vi "CreateScanPattern.vi"(3 "Point Spacing":dbl, 4 "Number of Points":u8, 5 "Pattern":T1(ring)) -> (0 "Radius":dbl, 1 "Y coordinates":dbl[](array[numeric]), 2 "X coordinates":dbl[](array[numeric]))   [LabVIEW 2011]
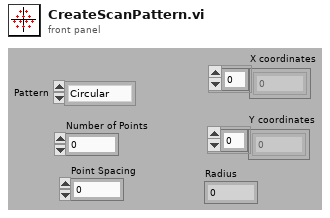
[diagram p1: front panel]
types:
  T1 = enum8{"Circular", "Square", "Hexagonal", "FilledSquare"}
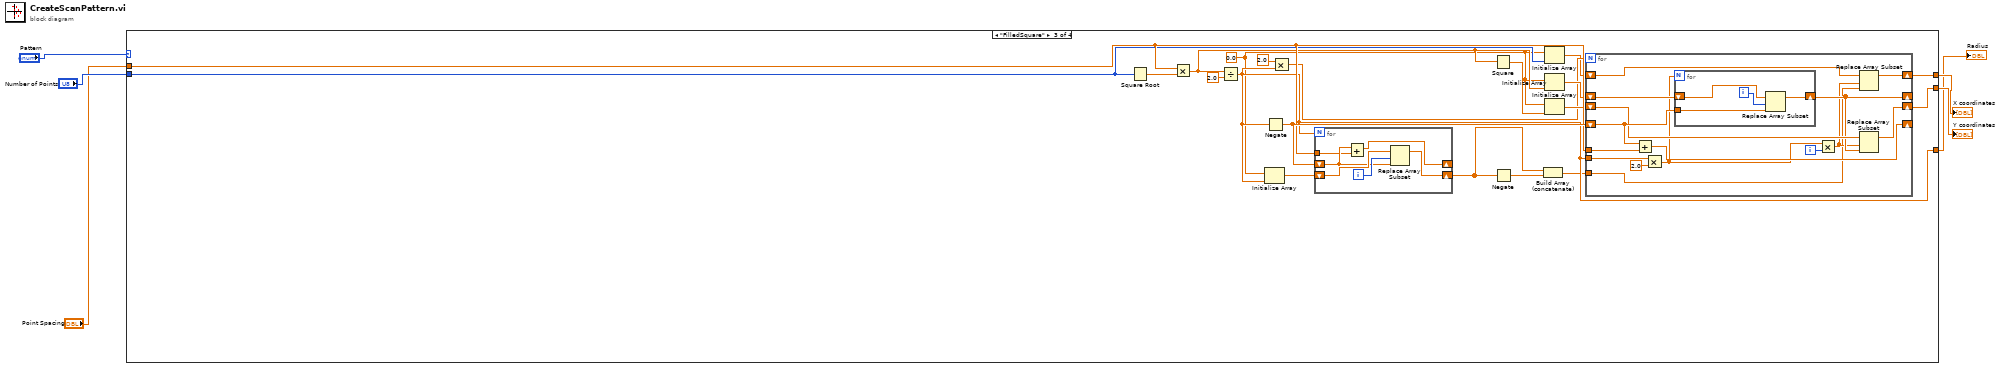
[diagram p0: block diagram]
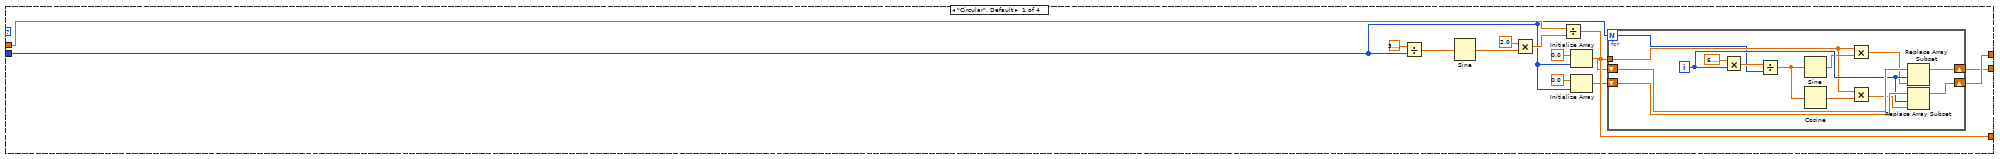
[diagram p2: hidden frame]
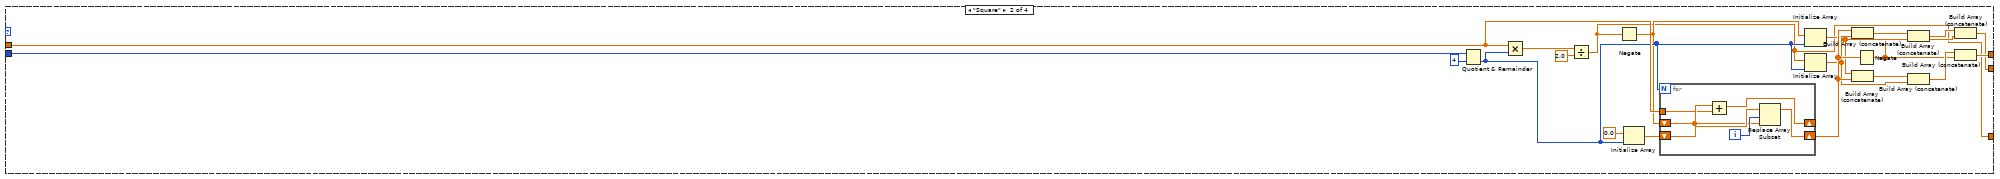
[diagram p3: hidden frame]
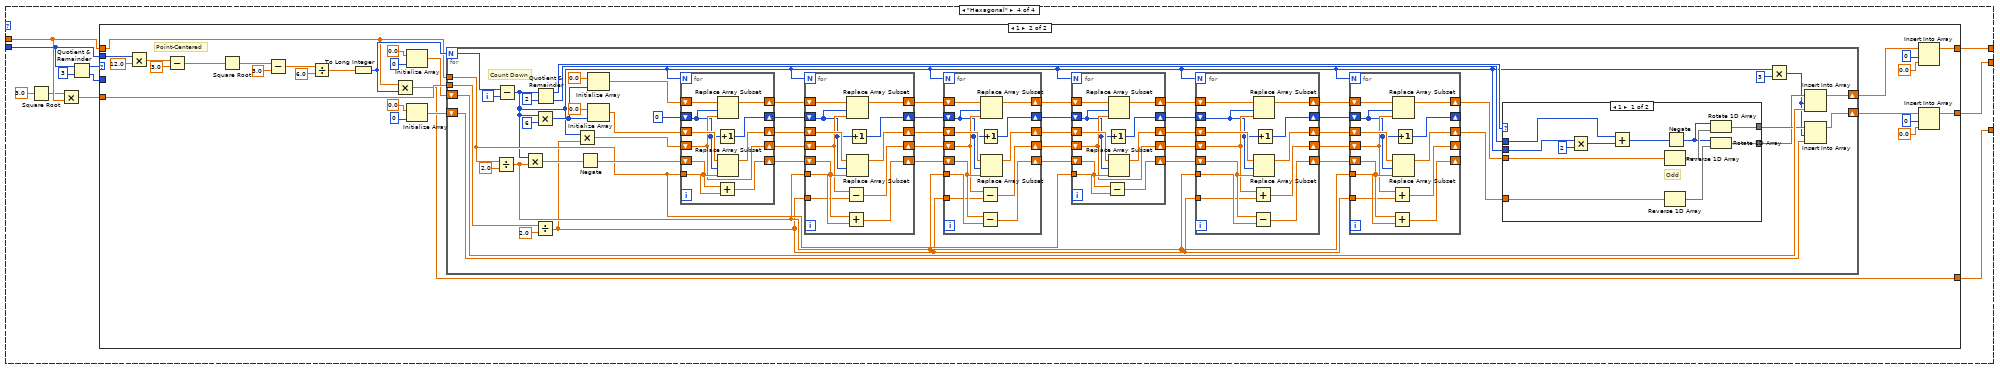
[diagram p4: hidden frame]
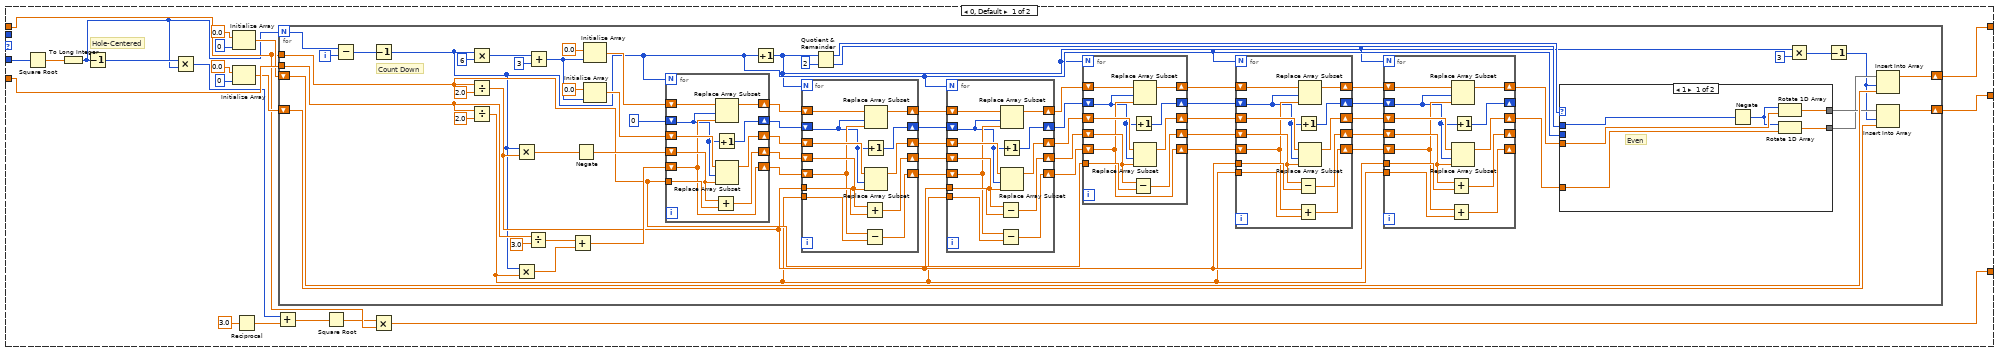
[diagram p5: hidden frame]
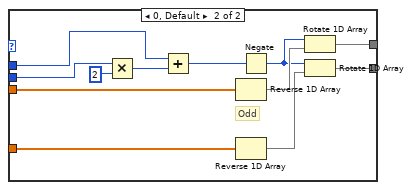
[diagram p6: hidden frame]
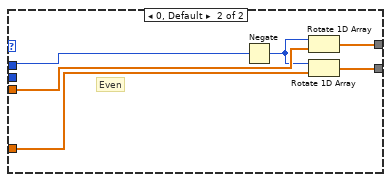
[diagram p7: hidden frame]
diagram:
  n1 = case shown="\"FilledSquare\"" "Pattern" {
    tunnel: "Point Spacing" -> [w15 w48 w75 w112]
    tunnel: "Number of Points" -> [w7 w54 w66 w107]
    tunnel: [w14 w43 w61 w109] -> w4
    tunnel: [w13 w40 w64 w108] -> w3
    tunnel: [w12 w35 w68 w106] -> w2
    frame "Circular", Default {
      n2 = Divide(x=3.141592653589793, y=w7) -> (x/y=w19:dbl)
      n3 = Sine(x=w19) -> (sin(x)=w18:dbl)
      n4 = Multiply(x=2.0, y=w18) -> (x*y=w16:dbl)
      n5 = Divide(x=w15, y=w16) -> (x/y=w12:dbl)
      n6 = Initialize Array(0.0 ("element"), w7) -> (w9:dbl[])
      n7 = Initialize Array(0.0 ("element"), w7) -> (w8:dbl[])
      n8 = for {
        N: w7 -> [w21]
        shift-right: [w28] -> w13
        shift-left: w9 -> [w33]
        shift-right: [w27] -> w14
        shift-left: w8 -> [w34]
        tunnel: w12 -> [w24]
        i -> [w32]
        n9 = Multiply(x=6.283185307179586, y=w32) -> (x*y=w30:dbl)
        n10 = Divide(x=w30, y=w21) -> (x/y=w29:dbl)
        n11 = Sine(x=w29) -> (sin(x)=w25:dbl)
        n12 = Cosine(x=w29) -> (cos(x)=w26:dbl)
        n13 = Multiply(x=w24, y=w25) -> (x*y=w23:dbl)
        n14 = Multiply(x=w24, y=w26) -> (x*y=w22:dbl)
        n15 = Replace Array Subset(array=w33, new element=w23, index=w32) -> (w28:dbl[])
        n16 = Replace Array Subset(array=w34, new element=w22, index=w32) -> (w27:dbl[])
      }
    }
    frame "Square" {
      n17 = Quotient & Remainder(x=w54, y=u8 4) -> (floor(x/y)=w47:u8)  [unwired: 1 out]
      n18 = Multiply(x=w48, y=w47) -> (x*y=w52:dbl)
      n19 = Divide(x=w52, y=2.0) -> (x/y=w35:dbl)
      n20 = Negate(x=w35) -> (-x=w46:dbl)
      n21 = Initialize Array(0.0 ("element"), w47) -> (w49:dbl[])
      n22 = for {
        N: w47 -> [_]
        shift-right: [w56] -> _
        shift-left: w46 -> [w58]
        shift-right: [w55] -> w39
        shift-left: w49 -> [w60]
        tunnel: w48 -> [w57]
        i -> [w59]
        n23 = Add(x=w58, y=w57) -> (x+y=w56:dbl)
        n24 = Replace Array Subset(array=w60, new element=w58, index=w59) -> (w55:dbl[])
      }
      n25 = Initialize Array(w46, w47) -> (w37:dbl[])
      n26 = Initialize Array(w35, w47) -> (w38:dbl[])
      n27 = Build Array (concatenate)(w39, w38) -> (w42:dbl[])
      n28 = Build Array (concatenate)(w37, w39) -> (w45:dbl[])
      n29 = Negate(x=w39) -> (-x=w36:dbl[])
      n30 = Build Array (concatenate)(w42, w36) -> (w41:dbl[])
      n31 = Build Array (concatenate)(w45, w38) -> (w44:dbl[])
      n32 = Build Array (concatenate)(w41, w37) -> (w40:dbl[])
      n33 = Build Array (concatenate)(w44, w36) -> (w43:dbl[])
    }
    frame "FilledSquare" {
      w65 = 0.0 ("element")
      n34 = Square Root(x=w66) -> (sqrt(x)=w79:dbl)
      n35 = Multiply(x=w75, y=w79) -> (x*y=w70:dbl)
      n36 = Divide(x=w70, y=2.0) -> (x/y=w68:dbl)
      n37 = Initialize Array(w65, w68) -> (w74:dbl[])
      n38 = Negate(x=w68) -> (-x=w76:dbl)
      n39 = Multiply(x=2.0, y=w68) -> (x*y=w67:dbl)
      n40 = for {
        N: w68 -> [_]
        shift-right: [w101] -> _
        shift-left: w76 -> [w103]
        shift-right: [w100] -> w78
        shift-left: w74 -> [w105]
        tunnel: w75 -> [w102]
        i -> [w104]
        n41 = Add(x=w103, y=w102) -> (x+y=w101:dbl)
        n42 = Replace Array Subset(array=w105, new element=w103, index=w104) -> (w100:dbl[])
      }
      n43 = Square(x=w70) -> (x^2=w71:dbl)
      n44 = Negate(x=w78) -> (-x=w77:dbl[])
      n45 = Build Array (concatenate)(w78, w77) -> (w62:dbl[])
      n46 = Initialize Array(w65, w66) -> (w63:dbl[])
      n47 = Initialize Array(w65, w70) -> (w73:dbl[])
      n48 = Initialize Array(w65, w71) -> (w72:dbl[])
      n49 = for {
        N: w67 -> [_]
        tunnel: w68 -> [w91]
        tunnel: w75 -> [w93]
        shift-right: [w94] -> _
        shift-left: w76 -> [w92]
        shift-right: [w87] -> _
        shift-left: w73 -> [w95]
        shift-right: [w88] -> w64
        shift-left: w72 -> [w89]
        shift-right: [w81] -> w61
        shift-left: w63 -> [w84]
        tunnel: w62 -> [w82]
        i -> [w85]
        n50 = Add(x=w92, y=w93) -> (x+y=w94:dbl)
        n51 = Multiply(x=w91, y=2.0) -> (x*y=w86:dbl)
        n52 = for {
          N: w86 -> [_]
          tunnel: w92 -> [w98]
          shift-right: [w96] -> w87
          shift-left: w95 -> [w97]
          i -> [w99]
          n53 = Replace Array Subset(array=w97, new element=w98, index=w99) -> (w96:dbl[])
        }
        n54 = Multiply(x=w86, y=w85) -> (x*y=w83:dbl)
        n55 = Replace Array Subset(array=w84, new element=w82, index=w83) -> (w81:dbl[])
        n56 = Replace Array Subset(array=w89, new element=w87, index=w83) -> (w88:dbl[])
      }
    }
    frame "Hexagonal" {
      n57 = Square Root(x=3.0) -> (sqrt(x)=w111:dbl)
      n58 = Multiply(x=w111, y=w112) -> (x*y=w113:dbl)
      n59 = Quotient & Remainder(x=w107, y=u8 3) -> (x-y*floor(x/y)=w115:u8, floor(x/y)=w110:u8)
      n60 = case shown="1" w115 {
        tunnel: w112 -> [w122 w289]
        tunnel: w113 -> [w130 w311]
        tunnel: w110 -> [w136 _]
        tunnel: [w127 w292] -> w109
        tunnel: [w126 w291] -> w108
        tunnel: w107 -> [_ w308]
        tunnel: [w121 w288] -> w106
        frame 0, Default {
          # "Hole-Centered"
          n61 = Square Root(x=w136) -> (sqrt(x)=w135:dbl)
          n62 = To Long Integer(number=w135) -> (32bit integer=w117:i32)
          n63 = Decrement(x=w117) -> (x-1=w118:i32)
          n64 = Multiply(x=w118, y=w117) -> (x*y=w125:i32)
          n65 = Initialize Array(0.0 ("element"), 0 ("dimension size")) -> (w129:dbl[])
          n66 = Initialize Array(0.0 ("element"), 0 ("dimension size")) -> (w128:dbl[])
          n67 = Reciprocal(x=3.0) -> (1/x=w124:dbl)
          n68 = Add(x=w125, y=w124) -> (x+y=w120:dbl)
          n69 = for {
            N: w117 -> [w155]
            tunnel: w122 -> [w172]
            tunnel: w130 -> [w185]
            shift-right: [w152] -> w127
            shift-left: w129 -> [w153]
            shift-right: [w151] -> w126
            shift-left: w128 -> [w149]
            i -> [w154]
            # "Count Down"
            n70 = Subtract(x=w155, y=w154) -> (x-y=w148:i32)
            n71 = Decrement(x=w148) -> (x-1=w141:i32)
            n72 = Multiply(x=w141, y=6) -> (x*y=w145:i32)
            n73 = Divide(x=w172, y=2.0) -> (x/y=w161:dbl)
            n74 = Divide(x=w185, y=2.0) -> (x/y=w160:dbl)
            n75 = Multiply(x=w141, y=w161) -> (x*y=w183:dbl)
            n76 = Multiply(x=w141, y=w160) -> (x*y=w186:dbl)
            n77 = Divide(x=w185, y=3.0) -> (x/y=w199:dbl)
            n78 = Add(x=w145, y=3) -> (x+y=w144:i32)
            n79 = Add(x=w199, y=w186) -> (x+y=w196:dbl)
            n80 = Negate(x=w183) -> (-x=w197:dbl)
            n81 = Initialize Array(0.0 ("element"), w144) -> (w192:dbl[])
            n82 = Initialize Array(0.0 ("element"), w144) -> (w193:dbl[])
            n83 = for {
              N: w141 -> [_]
              shift-right: [w280] -> w190
              shift-left: w197 -> [w283]
              shift-right: [w281] -> w188
              shift-left: w196 -> [w281]
              shift-right: [w286] -> w191
              shift-left: w193 -> [w287]
              shift-right: [w284] -> w189
              shift-left: w192 -> [w285]
              tunnel: w172 -> [w282]
              shift-right: [w278] -> w187
              shift-left: 0 ("y") -> [w279]
              n84 = Add(x=w283, y=w282) -> (x+y=w280:dbl)
              n85 = Increment(x=w279) -> (x+1=w278:i32)
              n86 = Replace Array Subset(array=w285, new element=w281, index=w279) -> (w284:dbl[])
              n87 = Replace Array Subset(array=w287, new element=w283, index=w279) -> (w286:dbl[])
            }
            n88 = Increment(x=w141) -> (x+1=w140:i32)
            n89 = for {
              N: w140 -> [_]
              shift-right: [w272] -> w180
              shift-left: w190 -> [w273]
              shift-right: [w268] -> w178
              shift-left: w188 -> [w270]
              shift-right: [w276] -> w181
              shift-left: w191 -> [w277]
              shift-right: [w274] -> w179
              shift-left: w189 -> [w275]
              tunnel: w161 -> [w271]
              shift-right: [w266] -> w182
              shift-left: w187 -> [w267]
              tunnel: w160 -> [w269]
              n90 = Add(x=w273, y=w271) -> (x+y=w272:dbl)
              n91 = Subtract(x=w270, y=w269) -> (x-y=w268:dbl)
              n92 = Increment(x=w267) -> (x+1=w266:i32)
              n93 = Replace Array Subset(array=w275, new element=w270, index=w267) -> (w274:dbl[])
              n94 = Replace Array Subset(array=w277, new element=w273, index=w267) -> (w276:dbl[])
            }
            n95 = Quotient & Remainder(x=w140, y=2) -> (x-y*floor(x/y)=w158:i32, floor(x/y)=w150:i32)
            n96 = for {
              N: w141 -> [_]
              shift-right: [w260] -> w175
              shift-left: w180 -> [w261]
              shift-right: [w257] -> w173
              shift-left: w178 -> [w258]
              shift-right: [w264] -> w176
              shift-left: w181 -> [w265]
              shift-right: [w262] -> w174
              shift-left: w179 -> [w263]
              tunnel: w161 -> [w259]
              shift-right: [w254] -> w177
              shift-left: w182 -> [w255]
              tunnel: w160 -> [w256]
              n97 = Subtract(x=w261, y=w259) -> (x-y=w260:dbl)
              n98 = Subtract(x=w258, y=w256) -> (x-y=w257:dbl)
              n99 = Increment(x=w255) -> (x+1=w254:i32)
              n100 = Replace Array Subset(array=w263, new element=w258, index=w255) -> (w262:dbl[])
              n101 = Replace Array Subset(array=w265, new element=w261, index=w255) -> (w264:dbl[])
            }
            n102 = for {
              N: w140 -> [_]
              shift-right: [w248] -> w169
              shift-left: w175 -> [w249]
              shift-right: [w246] -> w167
              shift-left: w173 -> [w246]
              shift-right: [w252] -> w170
              shift-left: w176 -> [w253]
              shift-right: [w250] -> w168
              shift-left: w174 -> [w251]
              tunnel: w172 -> [w247]
              shift-right: [w244] -> w171
              shift-left: w177 -> [w245]
              n103 = Subtract(x=w249, y=w247) -> (x-y=w248:dbl)
              n104 = Increment(x=w245) -> (x+1=w244:i32)
              n105 = Replace Array Subset(array=w251, new element=w246, index=w245) -> (w250:dbl[])
              n106 = Replace Array Subset(array=w253, new element=w249, index=w245) -> (w252:dbl[])
            }
            n107 = for {
              N: w141 -> [_]
              shift-right: [w238] -> w164
              shift-left: w169 -> [w239]
              shift-right: [w234] -> w162
              shift-left: w167 -> [w236]
              shift-right: [w242] -> w165
              shift-left: w170 -> [w243]
              shift-right: [w240] -> w163
              shift-left: w168 -> [w241]
              tunnel: w161 -> [w237]
              shift-right: [w232] -> w166
              shift-left: w171 -> [w233]
              tunnel: w160 -> [w235]
              n108 = Subtract(x=w239, y=w237) -> (x-y=w238:dbl)
              n109 = Add(x=w236, y=w235) -> (x+y=w234:dbl)
              n110 = Increment(x=w233) -> (x+1=w232:i32)
              n111 = Replace Array Subset(array=w241, new element=w236, index=w233) -> (w240:dbl[])
              n112 = Replace Array Subset(array=w243, new element=w239, index=w233) -> (w242:dbl[])
            }
            n113 = for {
              N: w140 -> [_]
              shift-right: [w226] -> _
              shift-left: w164 -> [w227]
              shift-right: [w222] -> _
              shift-left: w162 -> [w224]
              shift-right: [w230] -> w157
              shift-left: w165 -> [w231]
              shift-right: [w228] -> w156
              shift-left: w163 -> [w229]
              tunnel: w161 -> [w225]
              shift-right: [w220] -> _
              shift-left: w166 -> [w221]
              tunnel: w160 -> [w223]
              n114 = Add(x=w227, y=w225) -> (x+y=w226:dbl)
              n115 = Add(x=w224, y=w223) -> (x+y=w222:dbl)
              n116 = Replace Array Subset(array=w229, new element=w224, index=w221) -> (w228:dbl[])
              n117 = Replace Array Subset(array=w231, new element=w227, index=w221) -> (w230:dbl[])
              n118 = Increment(x=w221) -> (x+1=w220:i32)
            }
            n119 = case shown="1" w158 {
              tunnel: w157 -> [w205 w219]
              tunnel: w156 -> [w204 w218]
              tunnel: w141 -> [_ w214]
              tunnel: w150 -> [w203 w213]
              tunnel: [w207 w211] -> w146
              tunnel: [w206 w210] -> w147
              frame 1 {
                # "Even"
                n120 = Negate(x=w203) -> (-x=w202:i32)
                n121 = Rotate 1D Array(1:w204, 2:w202) -> (0:w206:dbl[])
                n122 = Rotate 1D Array(1:w205, 2:w202) -> (0:w207:dbl[])
              }
              frame 0, Default {
                # "Odd"
                n123 = Multiply(x=w214, y=2) -> (x*y=w215:i32)
                n124 = Add(x=w213, y=w215) -> (x+y=w209:i32)
                n125 = Reverse 1D Array(array=w218) -> (reversed array=w212:dbl[])
                n126 = Reverse 1D Array(array=w219) -> (reversed array=w217:dbl[])
                n127 = Negate(x=w209) -> (-x=w208:i32)
                n128 = Rotate 1D Array(1:w212, 2:w208) -> (0:w210:dbl[])
                n129 = Rotate 1D Array(1:w217, 2:w208) -> (0:w211:dbl[])
              }
            }
            n130 = Multiply(x=w140, y=3) -> (x*y=w138:i32)
            n131 = Decrement(x=w138) -> (x-1=w137:i32)
            n132 = Insert Into Array(array=w146, index=w137, new element=w153) -> (w152:dbl[])
            n133 = Insert Into Array(array=w147, index=w137, new element=w149) -> (w151:dbl[])
          }
          n134 = Square Root(x=w120) -> (sqrt(x)=w119:dbl)
          n135 = Multiply(x=w119, y=w122) -> (x*y=w121:dbl)
        }
        frame 1 {
          # "Point-Centered"
          n136 = Multiply(x=w308, y=12.0) -> (x*y=w306:dbl)
          n137 = Subtract(x=w306, y=3.0) -> (x-y=w304:dbl)
          n138 = Square Root(x=w304) -> (sqrt(x)=w303:dbl)
          n139 = Subtract(x=w303, y=3.0) -> (x-y=w301:dbl)
          n140 = Divide(x=w301, y=6.0) -> (x/y=w299:dbl)
          n141 = To Long Integer(number=w299) -> (32bit integer=w290:i32)
          n142 = Multiply(x=w289, y=w290) -> (x*y=w288:dbl)
          n143 = Initialize Array(0.0 ("element"), 0 ("dimension size")) -> (w310:dbl[])
          n144 = Initialize Array(0.0 ("element"), 0 ("dimension size")) -> (w309:dbl[])
          n145 = for {
            N: w290 -> [w330]
            tunnel: w289 -> [w347]
            tunnel: w311 -> [w360]
            shift-right: [w327] -> w294
            shift-left: w310 -> [w328]
            shift-right: [w326] -> w293
            shift-left: w309 -> [w324]
            i -> [w329]
            # "Count Down"
            n146 = Divide(x=w347, y=2.0) -> (x/y=w336:dbl)
            n147 = Subtract(x=w330, y=w329) -> (x-y=w318:i32)
            n148 = Multiply(x=w318, y=w336) -> (x*y=w358:dbl)
            n149 = Multiply(x=w318, y=6) -> (x*y=w320:i32)
            n150 = Divide(x=w360, y=2.0) -> (x/y=w335:dbl)
            n151 = Quotient & Remainder(x=w318, y=2) -> (x-y*floor(x/y)=w333:i32, floor(x/y)=w325:i32)
            n152 = Multiply(x=w318, y=w335) -> (x*y=w316:dbl)
            n153 = Negate(x=w358) -> (-x=w370:dbl)
            n154 = Initialize Array(0.0 ("element"), w320) -> (w366:dbl[])
            n155 = Initialize Array(0.0 ("element"), w320) -> (w367:dbl[])
            n156 = for {
              N: w318 -> [_]
              shift-right: [w451] -> w364
              shift-left: w370 -> [w454]
              shift-right: [w452] -> w362
              shift-left: w316 -> [w452]
              shift-right: [w457] -> w365
              shift-left: w367 -> [w458]
              shift-right: [w455] -> w363
              shift-left: w366 -> [w456]
              tunnel: w347 -> [w453]
              shift-right: [w449] -> w361
              shift-left: 0 ("y") -> [w450]
              n157 = Add(x=w454, y=w453) -> (x+y=w451:dbl)
              n158 = Increment(x=w450) -> (x+1=w449:i32)
              n159 = Replace Array Subset(array=w456, new element=w452, index=w450) -> (w455:dbl[])
              n160 = Replace Array Subset(array=w458, new element=w454, index=w450) -> (w457:dbl[])
            }
            n161 = for {
              N: w318 -> [_]
              shift-right: [w443] -> w355
              shift-left: w364 -> [w444]
              shift-right: [w439] -> w353
              shift-left: w362 -> [w441]
              shift-right: [w447] -> w356
              shift-left: w365 -> [w448]
              shift-right: [w445] -> w354
              shift-left: w363 -> [w446]
              tunnel: w336 -> [w442]
              shift-right: [w437] -> w357
              shift-left: w361 -> [w438]
              tunnel: w335 -> [w440]
              n162 = Subtract(x=w441, y=w440) -> (x-y=w439:dbl)
              n163 = Add(x=w444, y=w442) -> (x+y=w443:dbl)
              n164 = Replace Array Subset(array=w446, new element=w441, index=w438) -> (w445:dbl[])
              n165 = Replace Array Subset(array=w448, new element=w444, index=w438) -> (w447:dbl[])
              n166 = Increment(x=w438) -> (x+1=w437:i32)
            }
            n167 = for {
              N: w318 -> [_]
              shift-right: [w431] -> w350
              shift-left: w355 -> [w432]
              shift-right: [w428] -> w348
              shift-left: w353 -> [w429]
              shift-right: [w435] -> w351
              shift-left: w356 -> [w436]
              shift-right: [w433] -> w349
              shift-left: w354 -> [w434]
              tunnel: w336 -> [w430]
              shift-right: [w425] -> w352
              shift-left: w357 -> [w426]
              tunnel: w335 -> [w427]
              n168 = Subtract(x=w429, y=w427) -> (x-y=w428:dbl)
              n169 = Subtract(x=w432, y=w430) -> (x-y=w431:dbl)
              n170 = Increment(x=w426) -> (x+1=w425:i32)
              n171 = Replace Array Subset(array=w434, new element=w429, index=w426) -> (w433:dbl[])
              n172 = Replace Array Subset(array=w436, new element=w432, index=w426) -> (w435:dbl[])
            }
            n173 = for {
              N: w318 -> [_]
              shift-right: [w419] -> w344
              shift-left: w350 -> [w420]
              shift-right: [w417] -> w342
              shift-left: w348 -> [w417]
              shift-right: [w423] -> w345
              shift-left: w351 -> [w424]
              shift-right: [w421] -> w343
              shift-left: w349 -> [w422]
              tunnel: w347 -> [w418]
              shift-right: [w415] -> w346
              shift-left: w352 -> [w416]
              n174 = Subtract(x=w420, y=w418) -> (x-y=w419:dbl)
              n175 = Increment(x=w416) -> (x+1=w415:i32)
              n176 = Replace Array Subset(array=w422, new element=w417, index=w416) -> (w421:dbl[])
              n177 = Replace Array Subset(array=w424, new element=w420, index=w416) -> (w423:dbl[])
            }
            n178 = for {
              N: w318 -> [_]
              shift-right: [w409] -> w339
              shift-left: w344 -> [w410]
              shift-right: [w405] -> w337
              shift-left: w342 -> [w407]
              shift-right: [w413] -> w340
              shift-left: w345 -> [w414]
              shift-right: [w411] -> w338
              shift-left: w343 -> [w412]
              tunnel: w336 -> [w408]
              shift-right: [w403] -> w341
              shift-left: w346 -> [w404]
              tunnel: w335 -> [w406]
              n179 = Add(x=w407, y=w406) -> (x+y=w405:dbl)
              n180 = Subtract(x=w410, y=w408) -> (x-y=w409:dbl)
              n181 = Replace Array Subset(array=w412, new element=w407, index=w404) -> (w411:dbl[])
              n182 = Replace Array Subset(array=w414, new element=w410, index=w404) -> (w413:dbl[])
              n183 = Increment(x=w404) -> (x+1=w403:i32)
            }
            n184 = for {
              N: w318 -> [_]
              shift-right: [w397] -> _
              shift-left: w339 -> [w398]
              shift-right: [w393] -> _
              shift-left: w337 -> [w395]
              shift-right: [w401] -> w332
              shift-left: w340 -> [w402]
              shift-right: [w399] -> w331
              shift-left: w338 -> [w400]
              tunnel: w336 -> [w396]
              shift-right: [w391] -> _
              shift-left: w341 -> [w392]
              tunnel: w335 -> [w394]
              n185 = Add(x=w395, y=w394) -> (x+y=w393:dbl)
              n186 = Add(x=w398, y=w396) -> (x+y=w397:dbl)
              n187 = Replace Array Subset(array=w400, new element=w395, index=w392) -> (w399:dbl[])
              n188 = Replace Array Subset(array=w402, new element=w398, index=w392) -> (w401:dbl[])
              n189 = Increment(x=w392) -> (x+1=w391:i32)
            }
            n190 = case shown="1" w333 {
              tunnel: w332 -> [w384 w388]
              tunnel: w331 -> [w383 w387]
              tunnel: w318 -> [w379 _]
              tunnel: w325 -> [w378 w386]
              tunnel: [w376 w390] -> w322
              tunnel: [w375 w389] -> w323
              frame 1 {
                # "Odd"
                n191 = Multiply(x=w379, y=2) -> (x*y=w380:i32)
                n192 = Add(x=w378, y=w380) -> (x+y=w374:i32)
                n193 = Reverse 1D Array(array=w383) -> (reversed array=w377:dbl[])
                n194 = Reverse 1D Array(array=w384) -> (reversed array=w382:dbl[])
                n195 = Negate(x=w374) -> (-x=w373:i32)
                n196 = Rotate 1D Array(1:w377, 2:w373) -> (0:w375:dbl[])
                n197 = Rotate 1D Array(1:w382, 2:w373) -> (0:w376:dbl[])
              }
              frame 0, Default {
                # "Even"
                n198 = Negate(x=w386) -> (-x=w385:i32)
                n199 = Rotate 1D Array(1:w387, 2:w385) -> (0:w389:dbl[])
                n200 = Rotate 1D Array(1:w388, 2:w385) -> (0:w390:dbl[])
              }
            }
            n201 = Multiply(x=w318, y=3) -> (x*y=w319:i32)
            n202 = Insert Into Array(array=w322, index=w319, new element=w328) -> (w327:dbl[])
            n203 = Insert Into Array(array=w323, index=w319, new element=w324) -> (w326:dbl[])
          }
          n204 = Insert Into Array(array=w294, index=0, new element=0.0 ("new element/subarray")) -> (w292:dbl[])
          n205 = Insert Into Array(array=w293, index=0, new element=0.0 ("new element/subarray")) -> (w291:dbl[])
        }
      }
    }
  }
  "Radius" <- w2
  "X coordinates" <- w4
  "Y coordinates" <- w3
